vi "Real Inverse Matrix.vi"(2 "matrix type":T1, 3 "Input Matrix":T2) -> (0 "error":i32, 1 "Inverse Matrix":T2)   [LabVIEW 2020, in "NI_AALBase.lvlib"]
doc: "Finds <B>Inverse Matrix</B>, if it exists, of <B>Input Matrix</B>. Wire data to the <B>Input Matrix</B> input to determine the polymorphic instance to use or manually select the instance."
uses:
  NI_AALBase.lvlib
  RealMatrix.ctl
  Matrix Type of Inverse Matrix.ctl
  NI_Matrix.lvlib
panel:
  # "Inverse Matrix"
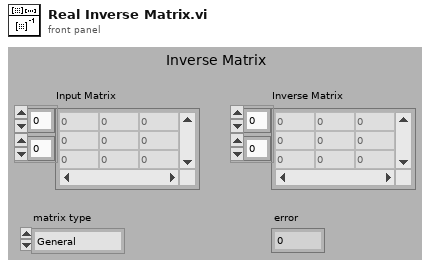
[diagram p1: front panel]
types:
  T1 = typedef "NI_AALBase.lvlib/Matrix Type of Inverse Matrix.ctl" = enum32{"General", "Positive Definite", "Lower Triangular", "Upper Triangular"}
  T2 = typedef "NI_Matrix.lvlib/RealMatrix.ctl" = dbl[][]
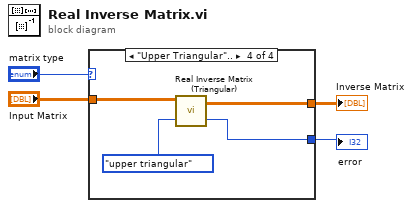
[diagram p0: block diagram]
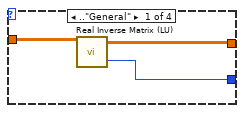
[diagram p2: hidden frame]
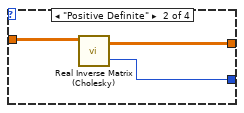
[diagram p3: hidden frame]
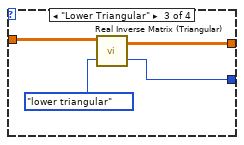
[diagram p4: hidden frame]
diagram:
  n1 = case shown="\"Upper Triangular\".." "matrix type" {
    tunnel: "Input Matrix" -> [w7 w8 w12 w16]
    tunnel: [w5 w9 w13 w17] -> w4
    tunnel: [w6 w10 w14 w18] -> w3
    frame .."General" {
      n2 = call "Real Inverse Matrix (LU).vi"("A"=w7) -> ("Inverse Matrix"=w6:T2, "error"=w5:i32)
    }
    frame "Positive Definite" {
      n3 = call "Real Inverse Matrix (Cholesky).vi"("A"=w8) -> ("Inverse Matrix"=w10:T2, "error"=w9:i32)
    }
    frame "Lower Triangular" {
      n4 = call "Real Inverse Matrix (Triangular).vi"("matrix type"=enum32{"lower triangular", "upper triangular"}."lower triangular", "A"=w12) -> ("error"=w13:i32, "Inverse Matrix"=w14:T2)
    }
    frame "Upper Triangular".. {
      n5 = call "Real Inverse Matrix (Triangular).vi"("matrix type"=enum32{"lower triangular", "upper triangular"}."upper triangular", "A"=w16) -> ("error"=w17:i32, "Inverse Matrix"=w18:T2)
    }
  }
  "Inverse Matrix" <- w3
  "error" <- w4
